vi "强度图2.vi"() -> ()   [LabVIEW 2012]
doc: "该范例演示了通过交互创建强度图色码表的方法。它可对Sine.vi生成的XY网格中的数据点计算强度值。第一次运行时将使用颜色映射。VI通过色码表允许用户创建新的色码表。"
panel:
  out "初始化的数组":dbl[][](array[numeric])
  in  "更改色码表 2":bool
  out "?":dbl[][](graph)
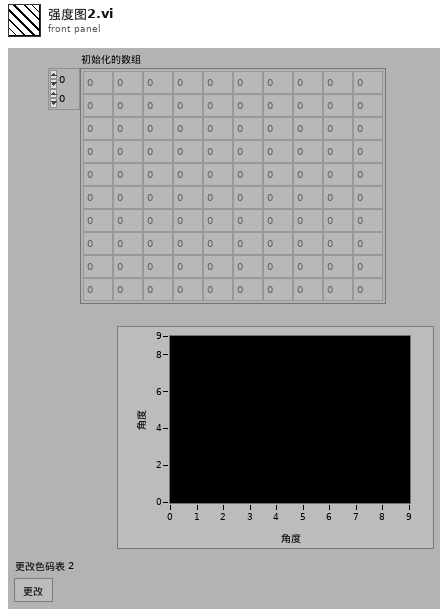
[diagram p1: front panel]
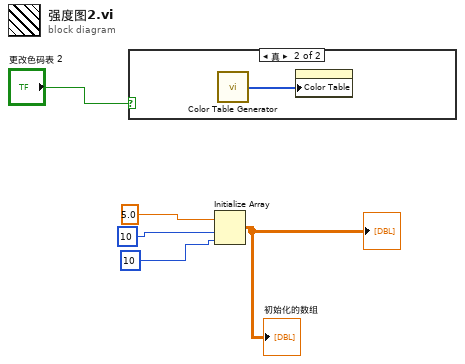
[diagram p0: block diagram]
diagram:
  n1 = case shown="真" "更改色码表 2" {
    frame False {
    }
    frame True {
      n2 = call "Color Table Generator.vi"() -> (w6:u32[])
      n3 = property class="IntGraph (严格)"("Color Table"=w6) -> ()  [unwired: 2 in, 2 out]
    }
  }
  n4 = Initialize Array(5.0 ("元素"), 10 ("维数大小"), 10 ("维数大小")) -> (→"?" →"初始化的数组":dbl[][])
